vi "hw6p3_hickey.vi"() -> ()   [LabVIEW 2014]
uses:
  <vilib>/Analysis/NI_AALPro.lvlib
panel:
  in  "# bins":i32
  in  "N":i32
  out "x histogram":T1(graph)
  out "Array":dbl[](array[numeric])
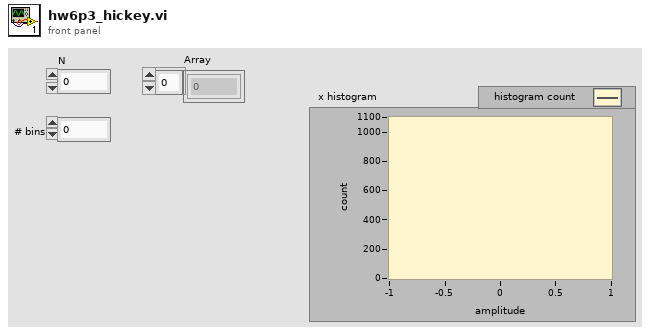
[diagram p1: front panel]
types:
  T1 = cluster{"X Values":dbl[], "Histogram: h(x)":i32[]}
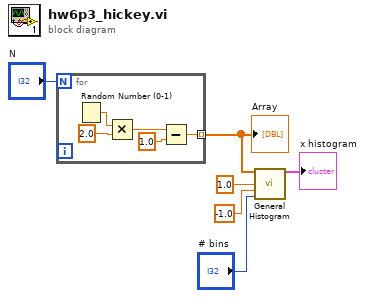
[diagram p0: block diagram]
diagram:
  n1 = for {
    N: "N" -> [_]
    tunnel: [w10] -> w5 mode=indexing
    n2 = Random Number (0-1)() -> (number: 0 to 1=w9:dbl)
    n3 = Multiply(x=w9, y=2.0) -> (x*y=w7:dbl)
    n4 = Subtract(x=w7, y=1.0) -> (x-y=w10:dbl)
  }
  "Array" <- w5
  n5 = call <vilib>:"General Histogram.vi"("X"=w5, "max"=1.0, "min"=-1.0, "# bins"="# bins") -> ("Histogram Graph"=→"x histogram":T1)  [unwired: 7 in, 4 out]
